vi "Gear Grab.vi"(11 "output cluster":T1) -> ()   [LabVIEW 2016]
uses:
  Joystick/ControlsToCommands.ctl
  <vilib>/Rock Robotics/WPI/Solenoid/WPI_SolenoidValue.ctl
  References/Refnums.vi
  <vilib>/Rock Robotics/WPI/Solenoid/WPI_SolenoidSetEnum.vi
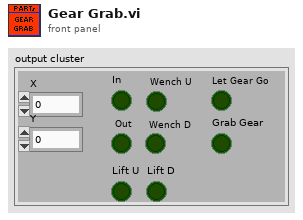
[diagram p1: front panel]
types:
  T1 = typedef "ControlsToCommands.ctl" = cluster{"X":dbl, "Y":dbl, "In":bool, " Out":bool, "Lift U":bool, " Wench U":bool, " Wench D":bool, "Lift D":bool, "Let Gear Go":bool, "Grab Gear":bool}
  T2 = typedef "WPI_SolenoidValue.ctl" = enum16{"Off", "On", "Forward", "Reverse"}
  T3 = typedef "WPI_SolenoidDevRef.ctl" = cluster{"DevStatus":errorcluster, "Pneumatics Control Module":u8, "Forward Solenoid Channel":T4, "Reverse Solenoid Channel":T4}
  T4 = typedef "WPI_SolenoidChannel.ctl" = enum8{"Solenoid 0", "Solenoid 1", "Solenoid 2", "Solenoid 3", "Solenoid 4", "Solenoid 5", "Solenoid 6", "Solenoid 7", "Invalid"}
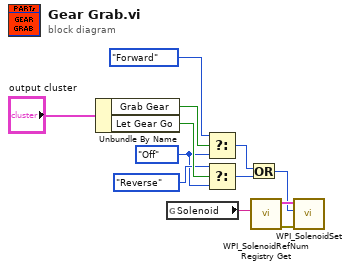
[diagram p0: block diagram]
diagram:
  w4 = WPI_SolenoidValue."Off" ("f")
  n1 = Unbundle By Name("output cluster") -> ("Grab Gear"=w8:bool, "Let Gear Go"=w6:bool)
  n2 = global read "Refnums.vi" "Solenoid"() -> (w11:string)
  n3 = Select(t=WPI_SolenoidValue."Forward" ("Value"), s=w8, f=w4) -> (s? t:f=w3:T2)
  n4 = Select(t=WPI_SolenoidValue."Reverse" ("Value"), s=w6, f=w4) -> (s? t:f=w2:T2)
  n5 = Or(x=w3, y=w2) -> (x .or. y?=w1:i32)
  n6 = call <vilib>:"WPI_SolenoidRefNum Registry Get.vi"("refnum name"=w11) -> ("error out"=w9:errorcluster, "SolenoidDevRef"=w10:T3)  [unwired: 9 in]
  n7 = call-poly <vilib>:"WPI_SolenoidSet.vi"("error in (no error)"=w9, "Value"=w1, "SolenoidDevRef"=w10) -> ()  [unwired: 7 in, 2 out]
